vi "fgt set pressure Limit.vi"(8 "error in (no error)":errorcluster, 9 "PlimMax":sgl, 10 "PlimMin":sgl, 11 "pressureIndex":u32) -> (0 "error out":errorcluster)   [LabVIEW 2020, in "fgt_SDK.lvlib"]
doc: "Set a limit, not to exceed on a pressure controller. It takes into account set unit, default value is 'mbar'.\nThis function is usefull when wanting to be sure not to go over a certain pressure value or during regulation.\nSetting a limit is used for next called functions. Limits can not exceed controller range."
uses:
  fgt_SDK.lvlib
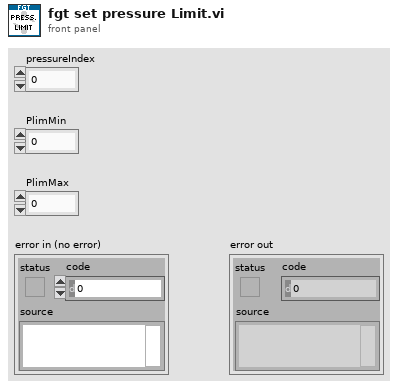
[diagram p1: front panel]
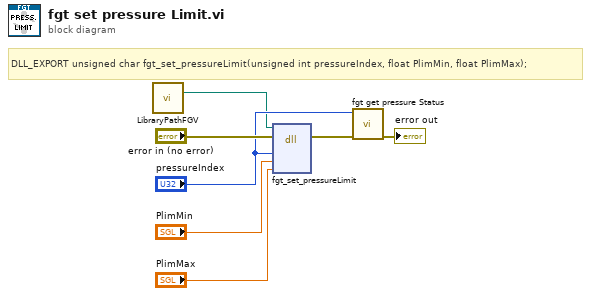
[diagram p0: block diagram]
diagram:
  # "DLL_EXPORT unsigned char fgt_set_pressureLimit(unsigned int pressureIndex, float PlimMin, float PlimMax);"
  n1 = call "LibraryPathFGV.vi"() -> ("Path Out"=w1:path)  [unwired: 14 in, 1 out]
  n2 = dll-call lib="C:/Workspace/fgt-SDK/LabVIEW/dlls/fgt_SDK_*.*" fn="fgt_set_pressureLimit"(path in=w1, error in="error in (no error)", "pressureIndex"="pressureIndex", "PlimMin"="PlimMin", "PlimMax"="PlimMax") -> (error out=w4:errorcluster)  [unwired: 5 in, 1 out]
  n3 = call "fgt get pressure Status.vi"("error in (no error)"=w4, "pressureIndex"="pressureIndex") -> ("error out"=→"error out":errorcluster)  [unwired: 9 in]
